vi "PQlistColumns.vi"(8 "error in":errorcluster, 10 "table":string, 11 "conn":u32) -> (0 "error out":errorcluster, 2 "Data":string[](array[string]), 3 "conn_out":u32)   [LabVIEW 2019, in "libpqutility.lvlib"]
uses:
  libpqutility.lvlib
  libpqlv/src/PQgetResult.vi
  libpqlv/src/PQclear.vi
  PQfetchTables.vi
  libpqlv/src/PQresultErrorMessage.vi
  libpqlv/src/PQresultStatus.vi
  libpqlv/src/PQsendQuery.vi
  libpqlv/src/PQgetvalue.vi
  libpqlv/src/PQntuples.vi
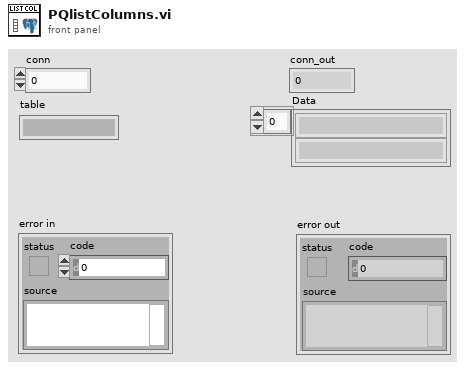
[diagram p1: front panel]
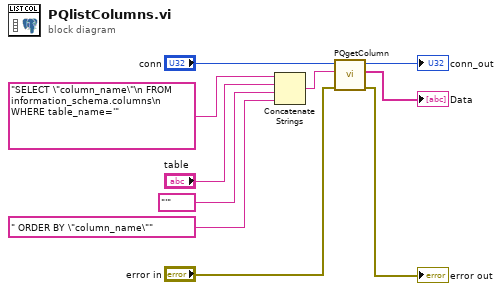
[diagram p0: block diagram]
diagram:
  n1 = Concatenate Strings("SELECT \"column_name\"\n FROM information_schema.columns\n WHERE table_name='" ("query"), "table", "'" ("query"), " ORDER BY \"column_name\"" ("query")) -> (w7:string)
  n2 = call "PQgetColumn.vi"("error in"="error in", "query"=w7, "conn"="conn") -> ("error out"=→"error out":errorcluster, "Data"=→"Data":string[], "conn_out"=→"conn_out":u32)  [unwired: 6 in]
